vi "MCS_SaveData.vi"(0 "Array":i32[](array[numeric]), 1 "Save File Name":string, 2 "Path":path) -> ()   [LabVIEW 2010]
uses:
  <vilib>/Utility/file.llb/Write To Spreadsheet File (I64).vi
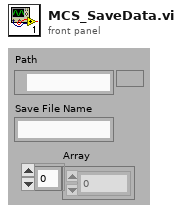
[diagram p1: front panel]
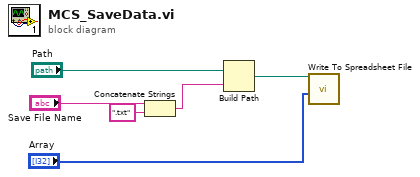
[diagram p0: block diagram]
diagram:
  n1 = Concatenate Strings("Save File Name", ".txt" ("string")) -> (w2:string)
  n2 = Build Path(base path="Path", name or relative path=w2) -> (appended path=w5:path)
  n3 = call-poly <vilib>:"Write To Spreadsheet File.vi"("1D data"="Array", "file path (dialog if empty)"=w5) -> ()  [unwired: 6 in, 1 out]
